vi "sv_Apply Fractional Octave Filter.vi"(0 "scaled signal [EU]":waveform(dbl), 5 "filter bank parameters":T1={"octave filter coefficients"=[{"filter structure"=enum."IIR 2nd Order", "Reverse Coefficients"=[1.0], "Forward Coefficients"=[]}], "lowpass filter coefficients"={"filter structure"=enum."IIR 2nd Order", "Reverse Coefficients"=[], "Forward Coefficients"=[]}, "number of samples to settle"=0, "number of decimation steps required"=[], "octave filter bandwidth"=[]}, 7 "internal filter state IN":T2, 9 "filter init/cont (init:F)":bool, 11 "error in (no error)":errorcluster) -> (4 "filtered data":waveform(dbl), 6 "dup filter bank parameters":T1={"octave filter coefficients"=[{"filter structure"=enum."IIR 2nd Order", "Reverse Coefficients"=[1.0], "Forward Coefficients"=[]}], "lowpass filter coefficients"={"filter structure"=enum."IIR 2nd Order", "Reverse Coefficients"=[], "Forward Coefficients"=[]}, "number of samples to settle"=0, "number of decimation steps required"=[], "octave filter bandwidth"=[]}, 8 "internal filter state OUT":T2, 10 "settled?":bool, 15 "error out":errorcluster)   [LabVIEW 2017, in "SoundVib_Octave_2014 standard.lvlib"]
doc: "This VI applies the designed single octave filter to input time domain signal.\n\nThe internal filter state IN and internal filter state OUT keep track of the internal state of the filter to ensure continuous operation of the filter. To achieve this continuous operation, you must call this VI the first time with filter init/cont set to FALSE. Call it all subsequent times with filter init/cont set to TRUE. Wire the internal filter state OUT of this call to the internal filter state IN for the next call to this VI."
uses:
  <vilib>/addons/Sound and Vibration/svt_Octave/SoundVib_Octave_2014 standard.lvlib
  <vilib>/addons/_NISVFA/_Shared subVIs/Controls/svc_Octave Filter Bank Parameters.ctl
  <vilib>/addons/_NISVFA/_Shared subVIs/Controls/svc_Octave Filter State.ctl
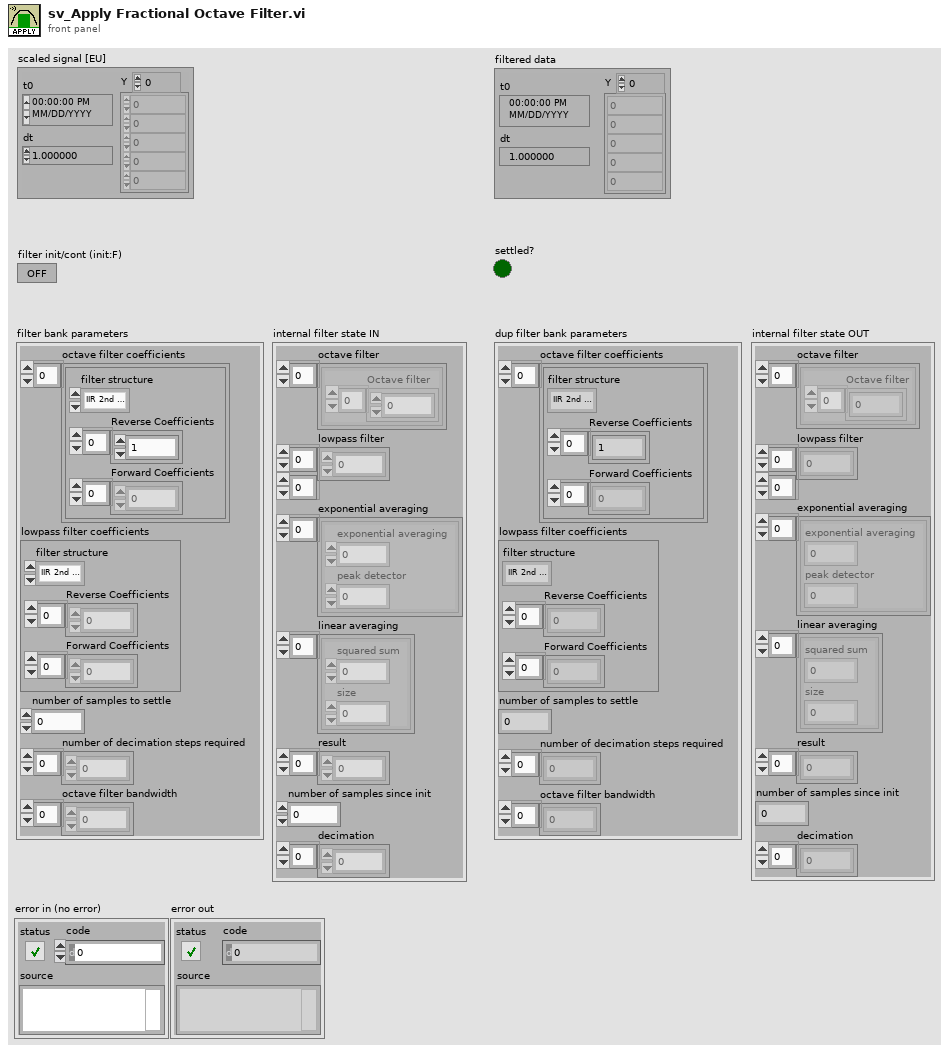
[diagram p1: front panel]
types:
  T1 = typedef "svc_Octave Filter Bank Parameters.ctl" = cluster{"octave filter coefficients":cluster{"filter structure":enum32{"IIR 2nd Order", "IIR 4th Order"}, "Reverse Coefficients":dbl[], "Forward Coefficients":dbl[]}[], "lowpass filter coefficients":cluster{"filter structure":enum32{"IIR 2nd Order", "IIR 4th Order"}, "Reverse Coefficients":dbl[], "Forward Coefficients":dbl[]}, "number of samples to settle":u64, "number of decimation steps required":i32[], "octave filter bandwidth":dbl[]}
  T2 = typedef "svc_Octave Filter State.ctl" = cluster{"octave filter":cluster{"Octave filter":dbl[]}[], "lowpass filter":dbl[][], "exponential averaging":cluster{"exponential averaging":dbl, "peak detector":dbl}[], "linear averaging":cluster{"squared sum":dbl, "size":dbl}[], "result":dbl[], "number of samples since init":u64, "decimation":dbl[]}
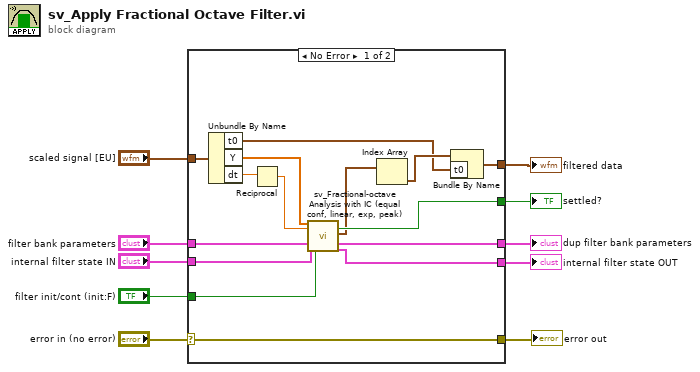
[diagram p0: block diagram]
diagram:
  n1 = case shown="No Error" "error in (no error)" {
    selector: "error in (no error)" -> [w13 w26]
    tunnel: "filter init/cont (init:F)" -> [w25 _]
    tunnel: [w24 _] -> w9
    tunnel: "scaled signal [EU]" -> [w23 _]
    tunnel: [w18 _] -> w7
    tunnel: "internal filter state IN" -> [w17 _]
    tunnel: "filter bank parameters" -> [w16 _]
    tunnel: [w15 _] -> w4
    tunnel: [w14 _] -> w3
    tunnel: [w13 w26] -> w1
    frame No Error {
      n2 = Unbundle By Name(w23) -> ("t0"=w19:timestamp, "Y"=w22:dbl[], "dt"=w12:dbl)
      n3 = Reciprocal(x=w12) -> (1/x=w11:dbl)
      n4 = call <vilib>:"sv_Fractional-octave Analysis with IC (equal conf, linear, exp, peak).vi"("scaled signal [EU]"=w22, "sampling frequency [Hz]"=w11, "filter bank parameters"=w16, "internal filter state IN"=w17, "filter init/cont (init:F)"=w25) -> ("settled?"=w24:bool, "filtered data array"=w21:waveform(dbl)[], "dup filter bank parameters"=w14:T1, "internal filter state OUT"=w15:T2)  [unwired: 10 in, 1 out]
      n5 = Index Array(array=w21) -> (element=w20:waveform(dbl))  [unwired: 1 in]
      n6 = Bundle By Name(cluster=w20, "t0"=w19) -> (w18:waveform(dbl))
    }
    frame Error {
    }
  }
  "settled?" <- w9
  "internal filter state OUT" <- w4
  "filtered data" <- w7
  "dup filter bank parameters" <- w3
  "error out" <- w1
